vi "Write File.vi"(8 "error in":errorcluster, 10 "Data In":refnum<class "Data.lvclass">, 11 "File Obs in":refnum<class "cCRDS File Obs.lvclass">) -> (0 "error out":errorcluster, 3 "File Obs out":refnum<class "cCRDS File Obs.lvclass">)   [LabVIEW 2015, in "cCRDS File Obs.lvclass"]
uses:
  cCRDS File Obs.lvclass
  Reusable/Data/Data.lvclass
  Reusable/CRDS/Data/Main/crd_data_enum.ctl
  CRDS/Data/cCRDS Data.lvclass
  Controls/MFC Address.ctl
  Reusable/File IO/Class/File Observer.lvclass/File Observer.ctl
  Reusable/File IO/Class/Read File Ref.vi
  CRDS/Data/Read vData.vi
  CRDS/Data/Read Humidifier T.vi
  Reusable/CRDS/File Observer/CRD File Obs.lvclass
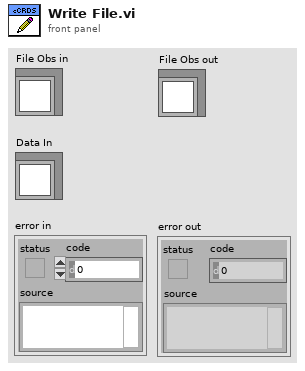
[diagram p1: front panel]
types:
  T1 = typedef "crd_data_enum.ctl" = enum8{"Time", "RHw", "TRH", "P", "Tmean", "RHsense", "TQ", "PQ", "Q", "Q0", "Qcal", "Qset", "extDilFac", "taucorr", "tau0corr", "stdevtau", "ext", "extCorr", "etau", "tau", "tau0", "Purge_Data", "NoData", "reserved", "Ttec", "Ang Exp", "Gamma", "filter", "fOverride", "notes", "max amp", "Tthermistor", "RhdilFac", "Psense", "TRHsense_bank", "RHsense_bank", "MFC_Data", "Thum", "ThumSP", "O3 Flow", "Pinlet Flow", "CLAP Flow", "O3 Add Valve", "O2 Valve", "O3 Cal"}
  T2 = typedef "MFC Address.ctl" = enum16{"CRDS Purge", "CRDS Thermodenuded", "CRDS Dry", "CRDS Med RH", "CRDS High RH", "PAS Ch 1", "PAS Ch 2", "PAS Ch3", "PAS Ch 4", "PAS Ch 5", "CLAP", "O3", "Pinlet"}
  T3 = enum16{"big-endian, network order", "native, host order", "little-endian"}
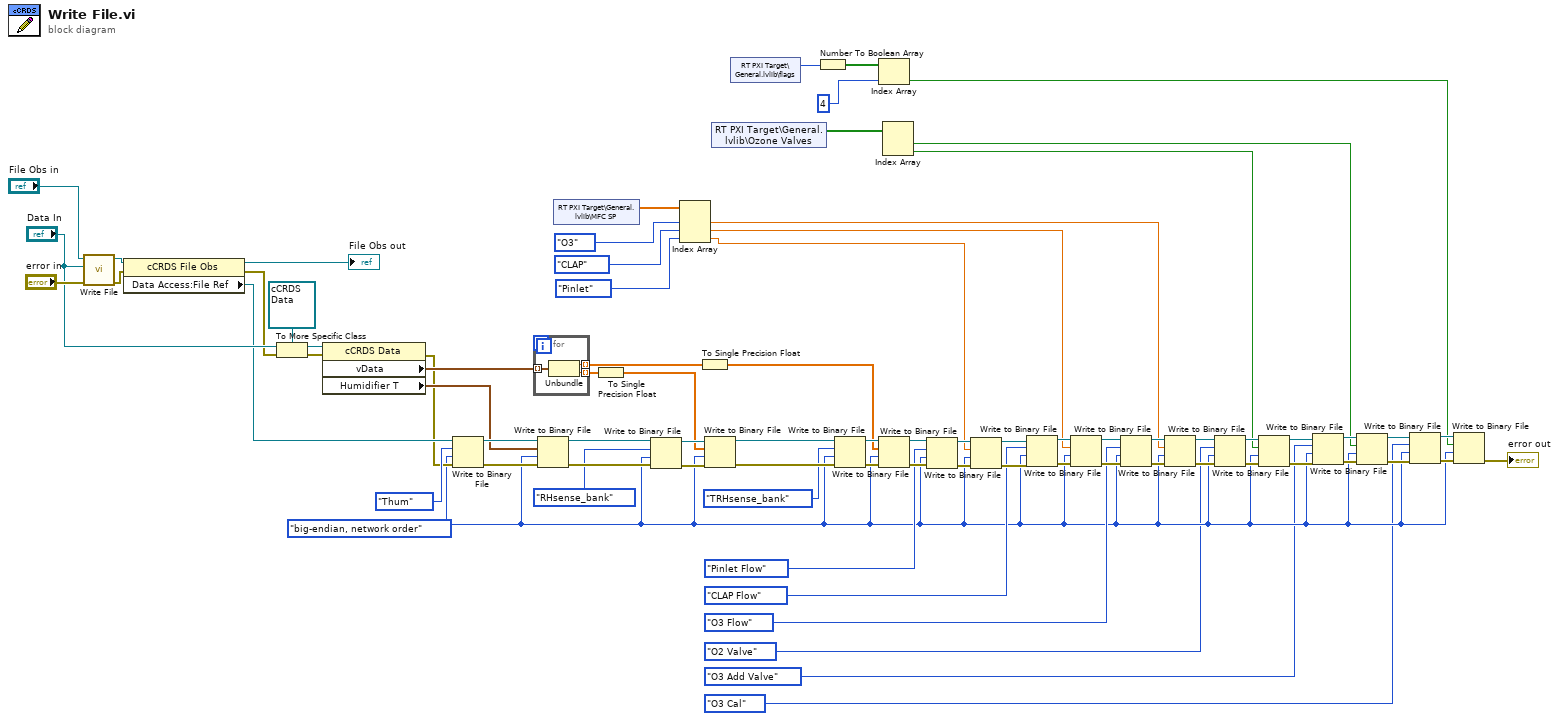
[diagram p0: block diagram]
diagram:
  w12 = T3."big-endian, network order" ("byte order (0:big-endian, network order)")
  n1 = call-parent "Write File.vi"("error in"="error in", "Data In"="Data In", "File Obs in"="File Obs in") -> ("error out"=w51:errorcluster, "File Obs out"=w52:refnum<class "cCRDS File Obs.lvclass">)  [unwired: 7 in]
  n2 = property class="cCRDS File Obs"(reference=w52, error in=w51) -> (reference out=→"File Obs out":refnum<class "cCRDS File Obs.lvclass">, error out=w49:errorcluster, "Data Access:File Ref"=w50:refnum<file>)
  n3 = To More Specific Class(target class=refnum<class "cCRDS Data.lvclass"> refnum ("cCRDS Data"), reference="Data In", error in=w49) -> (specific class reference=w58:refnum<class "cCRDS Data.lvclass">, error out=w53:errorcluster)
  n4 = property class="cCRDS Data"(reference=w58, error in=w53) -> (error out=w48:errorcluster, "vData"=w56:cluster{"TRH":dbl, "RH":dbl}[], "Humidifier T"=w57:cluster{"Hum 1":sgl, "Hum 2":sgl})  [unwired: 1 out]
  n5 = Write to Binary File(file (use dialog)=w50, data=crd_data_enum."Thum" ("CRD_Data_Enum"), error in=w48, 9:w12) -> (refnum out=w74:refnum<file>, error out=w73:errorcluster)  [unwired: 2 in, 1 out]
  n6 = for {
    tunnel: w56 -> [w80] mode=indexing
    tunnel: [w79] -> w55 mode=indexing
    tunnel: [w78] -> w54 mode=indexing
    n7 = Unbundle(w80) -> ("TRH"=w79:dbl, "RH"=w78:dbl)
  }
  n8 = Write to Binary File(file (use dialog)=w74, data=w57, error in=w73, 9:w12) -> (refnum out=w72:refnum<file>, error out=w71:errorcluster)  [unwired: 2 in, 1 out]
  n9 = shared-variable "RT PXI Target\\General.lvlib\\MFC SP"() -> (w46:sgl[])  [unwired: 1 in, 1 out]
  n10 = To Single Precision Float(number=w54) -> (single precision float=w67:sgl[])
  n11 = Write to Binary File(file (use dialog)=w72, data=crd_data_enum."RHsense_bank" ("CRD_Data_Enum"), error in=w71, 9:w12) -> (refnum out=w69:refnum<file>, error out=w68:errorcluster)  [unwired: 2 in, 1 out]
  n12 = Index Array(array=w46, index #1=MFC_Address."O3" ("Controllers"), index #2=MFC_Address."CLAP" ("Controllers"), index #3=MFC_Address."Pinlet" ("Controllers")) -> (element #1=w30:sgl, element #2=w29:sgl, element #3=w28:sgl)
  n13 = To Single Precision Float(number=w55) -> (single precision float=w61:sgl[])
  n14 = Write to Binary File(file (use dialog)=w69, data=w67, error in=w68, 9:w12) -> (refnum out=w66:refnum<file>, error out=w65:errorcluster)  [unwired: 2 in, 1 out]
  n15 = shared-variable "RT PXI Target\\General.lvlib\\Ozone Valves"() -> (w11:bool[])  [unwired: 1 in, 1 out]
  n16 = shared-variable "RT PXI Target\\General.lvlib\\flags"() -> (w6:u8)  [unwired: 1 in, 1 out]
  n17 = Number To Boolean Array(number=w6) -> (Boolean array=w5:bool[])
  n18 = Write to Binary File(file (use dialog)=w66, data=crd_data_enum."TRHsense_bank" ("CRD_Data_Enum"), error in=w65, 9:w12) -> (refnum out=w64:refnum<file>, error out=w63:errorcluster)  [unwired: 2 in, 1 out]
  n19 = Index Array(array=w5, index=4) -> (element=w3:bool)
  n20 = Write to Binary File(file (use dialog)=w64, data=w61, error in=w63, 9:w12) -> (refnum out=w39:refnum<file>, error out=w40:errorcluster)  [unwired: 2 in, 1 out]
  n21 = Index Array(array=w11) -> (element #1=w10:bool, element #2=w9:bool)  [unwired: 2 in]
  n22 = Write to Binary File(file (use dialog)=w39, data=crd_data_enum."Pinlet Flow" ("CRD_Data_Enum"), error in=w40, 9:w12) -> (refnum out=w41:refnum<file>, error out=w42:errorcluster)  [unwired: 2 in, 1 out]
  n23 = Write to Binary File(file (use dialog)=w41, data=w28, error in=w42, 9:w12) -> (refnum out=w35:refnum<file>, error out=w36:errorcluster)  [unwired: 2 in, 1 out]
  n24 = Write to Binary File(file (use dialog)=w35, data=crd_data_enum."CLAP Flow" ("CRD_Data_Enum"), error in=w36, 9:w12) -> (refnum out=w38:refnum<file>, error out=w37:errorcluster)  [unwired: 2 in, 1 out]
  n25 = Write to Binary File(file (use dialog)=w38, data=w29, error in=w37, 9:w12) -> (refnum out=w31:refnum<file>, error out=w32:errorcluster)  [unwired: 2 in, 1 out]
  n26 = Write to Binary File(file (use dialog)=w31, data=crd_data_enum."O3 Flow" ("CRD_Data_Enum"), error in=w32, 9:w12) -> (refnum out=w33:refnum<file>, error out=w34:errorcluster)  [unwired: 2 in, 1 out]
  n27 = Write to Binary File(file (use dialog)=w33, data=w30, error in=w34, 9:w12) -> (refnum out=w21:refnum<file>, error out=w22:errorcluster)  [unwired: 2 in, 1 out]
  n28 = Write to Binary File(file (use dialog)=w21, data=crd_data_enum."O2 Valve" ("CRD_Data_Enum"), error in=w22, 9:w12) -> (refnum out=w24:refnum<file>, error out=w23:errorcluster)  [unwired: 2 in, 1 out]
  n29 = Write to Binary File(file (use dialog)=w24, data=w9, error in=w23, 9:w12) -> (refnum out=w17:refnum<file>, error out=w18:errorcluster)  [unwired: 2 in, 1 out]
  n30 = Write to Binary File(file (use dialog)=w17, data=crd_data_enum."O3 Add Valve" ("CRD_Data_Enum"), error in=w18, 9:w12) -> (refnum out=w19:refnum<file>, error out=w20:errorcluster)  [unwired: 2 in, 1 out]
  n31 = Write to Binary File(file (use dialog)=w19, data=w10, error in=w20, 9:w12) -> (refnum out=w14:refnum<file>, error out=w13:errorcluster)  [unwired: 2 in, 1 out]
  n32 = Write to Binary File(file (use dialog)=w14, data=crd_data_enum."O3 Cal" ("CRD_Data_Enum"), error in=w13, 9:w12) -> (refnum out=w16:refnum<file>, error out=w15:errorcluster)  [unwired: 2 in, 1 out]
  n33 = Write to Binary File(file (use dialog)=w16, data=w3, error in=w15, 9:w12) -> (error out=→"error out":errorcluster)  [unwired: 2 in, 2 out]
